vi "HFLI_sys_test.vi"() -> ()   [LabVIEW 2015]
uses:
  KM_ControlHFLIcommand.ctl
  KM_SystemParameters.ctl
panel:
  out "Plot: All":cluster{"all rows":dbl[], "all rows":dbl[]}[](graph)
  in  "ZI HFLI System Parameters IN":T1={"IP Address"="DEV987", "Start (Hz)"=10000.0, "Stop (Hz)"=1000000.0, "Filter Order"=4, "Number of Points"=100, "Precision"=0, "Bandwidth (Hz)"=-1.0, "Averaging"=1, "Log Sweep"=FALSE, "Vz Demod"=3, "Iz Demod"=1} {"Averaging" items=["1"=1, "2"=2, "4"=4, "16"=16, "32"=32, "64"=64]; "Bandwidth (Hz)" format="%#_p"; "Precision" items=["Low", "Med", "High"]; "Number of Points" min=2 max=66000; "Filter Order" items=["6, 1st"=1, "12, 2nd"=2, "18, 3rd"=3, "24, 4th"=4, "30, 5th"=5, "36, 6th"=6, "42, 7th"=7, "48, 8th"=8]; "Stop (Hz)" format="%_5p"; "Start (Hz)" format="%_5p"}
  in  "Control HFLI command":T2=enum."Scan frequency"
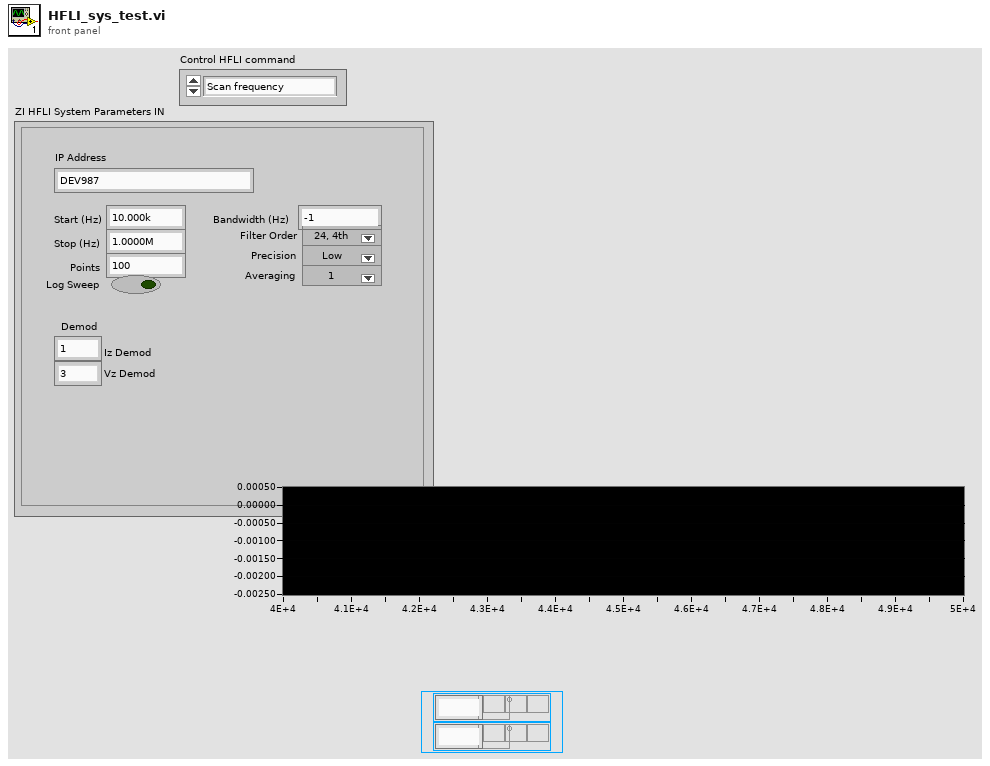
[diagram p1: front panel]
types:
  T1 = typedef "KM_SystemParameters.ctl" = cluster{"IP Address":string, "Start (Hz)":dbl, "Stop (Hz)":dbl, "Filter Order":i32, "Number of Points":i32, "Precision":u16, "Bandwidth (Hz)":dbl, "Averaging":u16, "Log Sweep":bool, "Vz Demod":i32, "Iz Demod":i32}
  T2 = typedef "KM_ControlHFLIcommand.ctl" = enum16{"Initialize", "Scan frequency"}
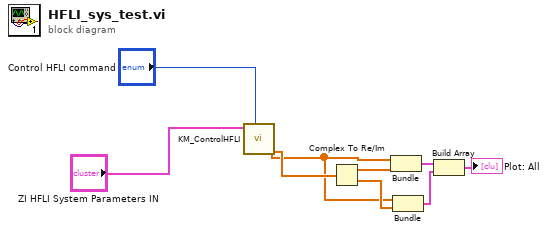
[diagram p0: block diagram]
diagram:
  n1 = call "KM_ControlHFLI.vi"("Control HFLI command"="Control HFLI command", "ZI HFLI System Parameters IN"="ZI HFLI System Parameters IN") -> ("Voltage out"=w3:cdb[], "Freq out"=w1:dbl[])  [unwired: 5 in, 1 out]
  n2 = Complex To Re/Im(x + iy=w3) -> (x=w5:dbl[], y=w4:dbl[])
  n3 = Bundle("Freq out"=w1, w5) -> (w6:cluster{"Freq out":dbl[], dbl[]})  [unwired: 1 in]
  n4 = Bundle("Freq out"=w1, w4) -> (w2:cluster{"Freq out":dbl[], dbl[]})  [unwired: 1 in]
  n5 = Build Array(w6, w2) -> (→"Plot: All":cluster{"Freq out":dbl[], dbl[]}[])
